vi "Njord Control System.vi"() -> ()   [LabVIEW 2014]
doc: "The main VI"
uses:
  Supervisor/Supervisor.lvclass
  <vilib>/Platform/TimedLoop/XDataNode/timing_clust.ctl
  <vilib>/Platform/TimedLoop/XDataNode/nitl_modes.ctl
  <vilib>/Platform/TimedLoop/XDataNode/wakeup.ctl
  ROV/Vessel(TCPrefs).vi
  <vilib>/FPGAPlugInAG/cRIO-9074/niLvFpga_Open_cRIO-9074.vi
  ROV/Vessel(FPGARef).vi
  Supervisor/Supervisor().vi
  Library/Helping Routines/ReconnectProcedureScalar.vi
  <vilib>/rvi/interface/nirviOpenFPGA/nirviOpenFPGA.xnode
  FPGA Bitfiles/MinervaControlSy_FPGATarget_9870InterfaceDMA_4D1233B8.lvbitx
  cRIO/FPGA/9870 Interface DMA (FPGA).vi
  <vilib>/Platform/TimedLoop/XDataNode/XDataNode.xnode
  Thruster/Thruster.lvclass
  ROV/Vessel.lvclass
  <vilib>/Platform/TimedLoop/XDataNode/XDNodeRunTimeDep.lvlib
  Thrust Allocation/Thrust Allocation.lvclass
panel:
  in  "Recieve UDP PSIMSSB":u16=5113
  in  "Recieve UDP GPGGA":u16=5111
  in  "Recieve Navipac TCP Port":u16=5104
  in  "Recieve ROV TCP Port":u16=5102
  in  "Send Telebuf TCP Port":u16=5100
  in  "Communication control":bool=TRUE
  in  "UDP port":u16=1118
  out "remote address TCP joyst":string
  out "remote address TCP send 1":string
  out "remote address TCP recv":string
  in  "Ignore Semaphore\nTCP Send":bool=TRUE
  in  "Period TCP Thread":i64=50
  out "MainThread timed out":bool
  in  "Main\nTimeOut Limit":i32=-1
  in  "TCP Recv\nTimeOut Limit":i32=25
  in  "TCP Send\nTimeOut Limit":i32=25
  in  "TCP Joyst. \nTimeOut Limit":i32=15
  out "Error TCP Recv":errorcluster
  out "Error TCP Joystick":errorcluster
  out "Error TCP Send":errorcluster
  out "Error MainThread":errorcluster
  in  "Base Port Send TCP":u16=8500
  in  "Port Recv TCP":u16=8510
  in  "Port Joyst.TCP":u16=8520
  out "TCP Joyst. Iteration Duration":u32
  out "TCP Recv Iteration Duration":u32
  out "TCP Recv timed out":bool
  out "TCP Joystick timed out":bool
  out "TCP Send timed out":bool
  out "TCP Send Iteration Duration":i64
  out "TCP Send\nFinished Late?":bool
  out "Main Iteration Duration":i64
  out "Main Thread\nFinished Late?":bool
  out "Exit Error":errorcluster
  in  "Cancel Button":bool
  out "Supervisor":refnum<class "Supervisor.lvclass">
  # "Njord"
  # "cRIO/FPGA"
  # "TCP"
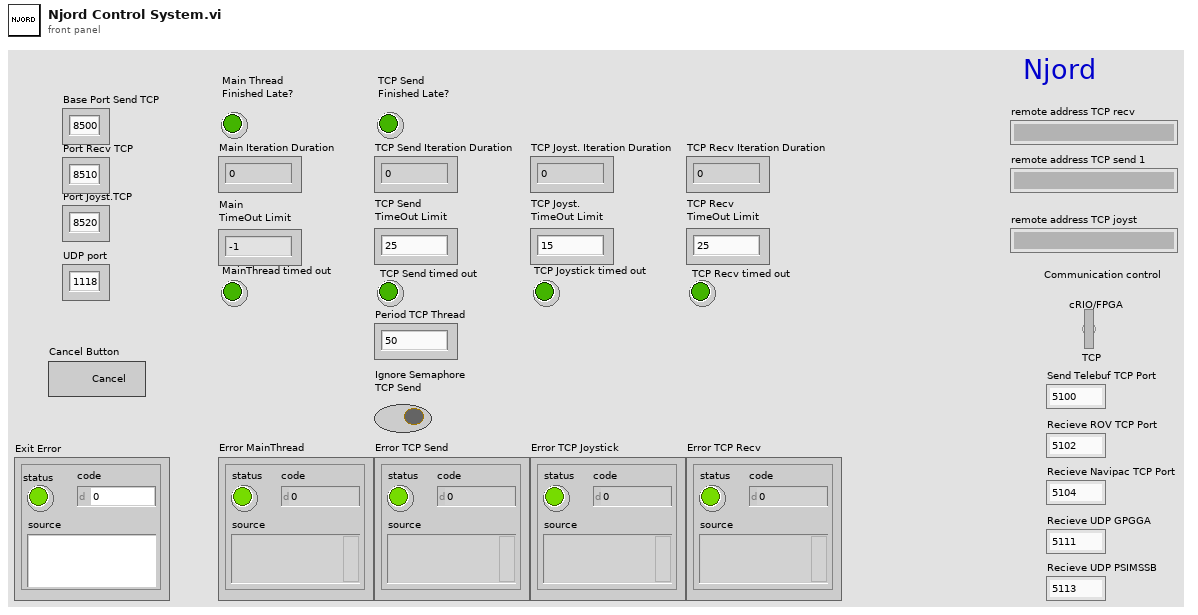
[diagram p1: front panel]
types:
  T1 = typedef "XDNodeRunTimeDep.lvlib/timing_clust.ctl" = cluster{"Expected End [f-1]":u64, "Actual End [f-1]":u64, "Finished Late? [f-1]":bool, "Expected End [i-1]":u64, "Actual End [i-1]":u64, "Finished Late? [i-1]":bool, "Expected Start [i]":u64, "Actual Start [i]":u64, "Expected Start [f]":u64, "Actual Start [f]":u64, "Source Name":string, "Structure Name":string, "Period":i64, "Deadline":i64, "Offset":i64, "Start":i64, "Priority":i32, "Timeout":i32, "Mode":T2, "Wakeup Reason":T3, "Error":errorcluster, "Source Type":string, "Secondary Source Type":string, "Global End Time":u64, "Global Start Time":u64, "Frame Duration":u64, "Iteration Duration":u64, "Assigned CPU":i32, "I/O Scan Engine Mode":u32}
  T2 = typedef "XDNodeRunTimeDep.lvlib/nitl_modes.ctl" = enum32{"No Change", "Process missed periods, maintain original phase", "Discard missed periods, maintain original phase", "Process missed periods, ignore original phase", "Discard missed periods, ignore original phase"}
  T3 = typedef "XDNodeRunTimeDep.lvlib/wakeup.ctl" = enum32{"Normal", "Aborted", "Asynchronous wakeup", "Timing source error", "Timed loop error", "Timeout"}
  T4 = typedef "Semaphore RefNum" = refnum<k1>
  T5 = typedef "Rendezvous RefNum" = refnum<k1>
  T6 = cluster{"Controllers":string[], "Observers":string[]}
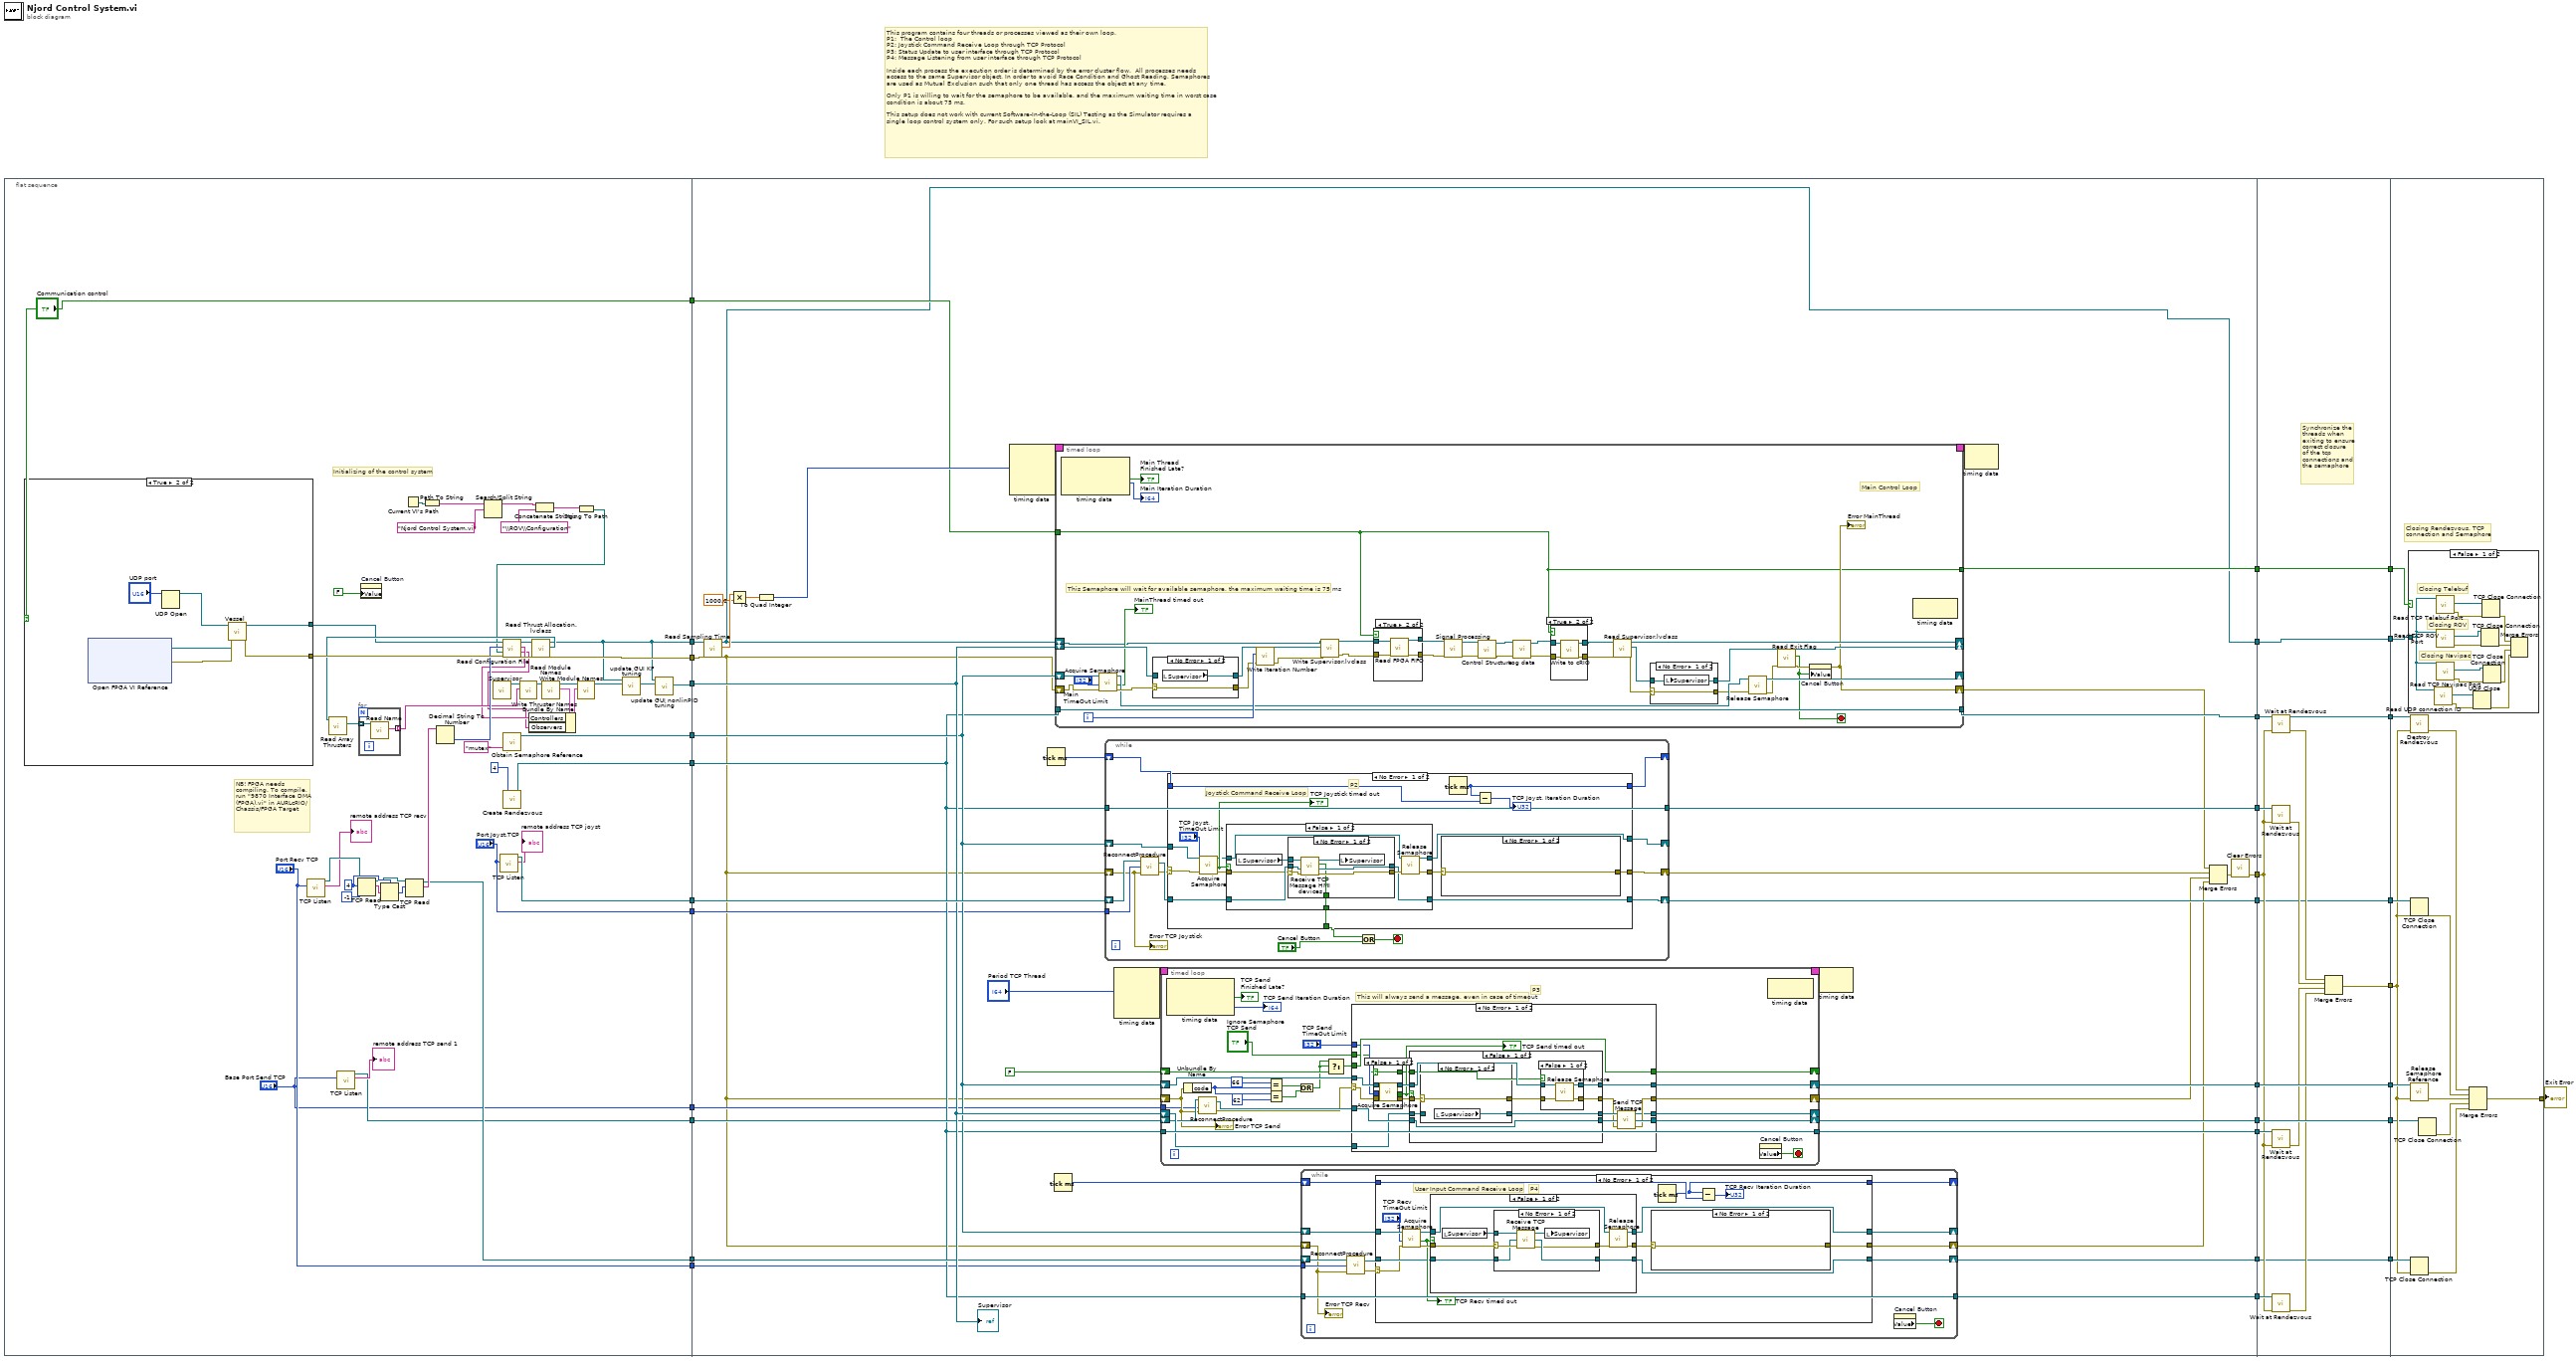
[diagram p0: block diagram]
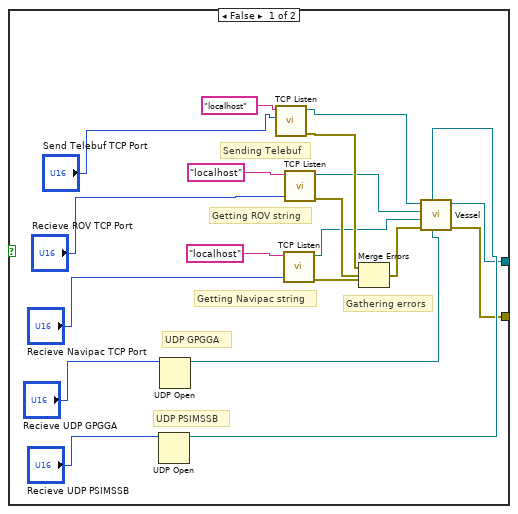
[diagram p2: hidden frame]
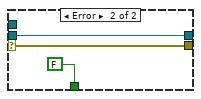
[diagram p3: hidden frame]
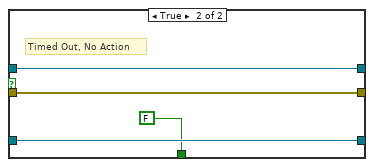
[diagram p4: hidden frame]
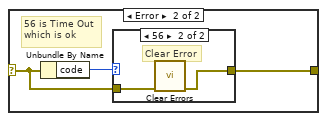
[diagram p5: hidden frame]
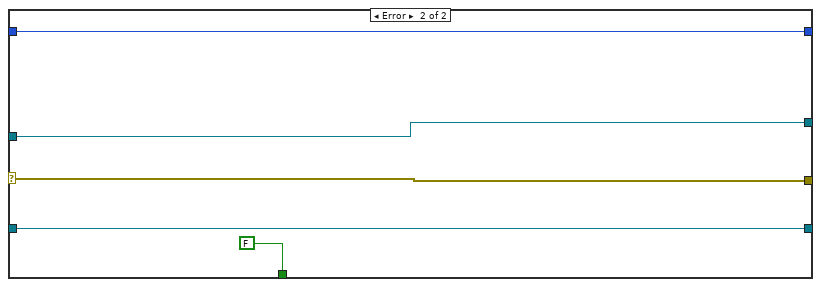
[diagram p7: hidden frame]
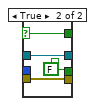
[diagram p8: hidden frame]
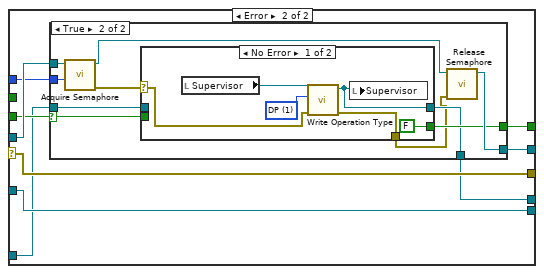
[diagram p12: hidden frame]
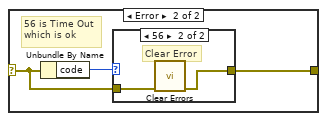
[diagram p15: hidden frame]
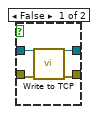
[diagram p20: hidden frame]
diagram:
  # "This program contains four threads or processes viewed as their own loop.\nP1:  The Control loop\nP2: Joystick Command Receive Loop through TCP Protocol\nP3: Status Update to user interface through TCP Protocol\nP4: Message Listening from user interface through TCP Protocol\n\nInside each process the execution order is determined by the error cluster flow.  All processes needs \naccess to the same Supervisor object. In order to avoid Race Condition and Ghost Reading, Semaphores\nare used as Mutual Exclusion such that only one thread has access the object at any time. \n\nOnly P1 is willing to wait for the semaphore to be available, and the maximum waiting time in worst case \ncondition is about 75 ms. \n\nThis setup does not work with current Software-In-the-Loop (SIL) Testing as the Simulator requires a\nsingle loop control system only. For such setup look at mainVI_SIL.vi."
  n1 = flat-sequence {
    tunnel: [w34] -> w32
    tunnel: [w53] -> w31
    tunnel: [w35] -> w30
    tunnel: [w69] -> w29
    tunnel: [w67] -> w28
    tunnel: [w80] -> w27
    tunnel: [w60] -> w22
    tunnel: [w77] -> w16
    tunnel: ["Port Joyst.TCP"] -> w7
    tunnel: ["Base Port Send TCP"] -> w6
    tunnel: ["Port Recv TCP"] -> w5
    tunnel: ["Communication control"] -> w4
    tunnel: w32 -> [w141]
    tunnel: w31 -> [w140]
    tunnel: w30 -> [w139]
    tunnel: w29 -> [w138]
    tunnel: w28 -> [w147]
    tunnel: w27 -> [w136]
    tunnel: [w115] -> w26
    tunnel: [w146] -> w25
    tunnel: [w145] -> w24
    tunnel: [w144] -> w23
    tunnel: w22 -> [w137]
    tunnel: [w135] -> w21
    tunnel: w16 -> [w134]
    tunnel: [w133] -> w15
    tunnel: [w132] -> w14
    tunnel: [w131] -> w13
    tunnel: [w130] -> w12
    tunnel: [w119] -> w10
    tunnel: w7 -> [w123]
    tunnel: w6 -> [w122]
    tunnel: w5 -> [w121]
    tunnel: w4 -> [w117]
    tunnel: [w116] -> w2
    tunnel: w26 -> [w461]
    tunnel: w25 -> [w463]
    tunnel: w24 -> [w475]
    tunnel: w23 -> [w476]
    tunnel: w21 -> [w464]
    tunnel: [w463] -> w20
    tunnel: [w476] -> w19
    tunnel: [w475] -> w18
    tunnel: [w464] -> w17
    tunnel: w15 -> [w474]
    tunnel: w14 -> [w473]
    tunnel: w13 -> [w471]
    tunnel: w12 -> [w472]
    tunnel: [w470] -> w11
    tunnel: w10 -> [w469]
    tunnel: [w462] -> w9
    tunnel: [w461] -> w3
    tunnel: w2 -> [w460]
    tunnel: [w460] -> w1
    tunnel: w20 -> [w490]
    tunnel: w19 -> [w489]
    tunnel: w18 -> [w480]
    tunnel: w17 -> [w488]
    tunnel: w11 -> [w487]
    tunnel: w9 -> [w486]
    tunnel: [w481] -> w8
    tunnel: w3 -> [w478]
    tunnel: w1 -> [w477]
    frame #0 {
      w74 = 4 ("bytes to read")
      # "Initializing of the control system"
      # "NB! FPGA needs compiling. To compile, run \"9870 Interface DMA (FPGA).vi\" in AURLcRIO/Chassis/FPGA Target"
      n2 = case shown="True" "Communication control" {
        tunnel: [w83 w106] -> w79
        tunnel: [w82 w101] -> w45
        frame False {
          # "UDP PSIMSSB"
          # "UDP GPGGA"
          # "Gathering errors"
          # "Sending Telebuf"
          # "Getting Navipac string"
          # "Getting ROV string"
          n3 = UDP Open(11:"Recieve UDP PSIMSSB") -> (port=w86:refnum<k16>)  [unwired: 4 in, 2 out]
          n4 = UDP Open(11:"Recieve UDP GPGGA") -> (port=w85:refnum<k16>)  [unwired: 4 in, 2 out]
          n5 = call <vilib>:"TCP Listen.vi"("port"="Send Telebuf TCP Port", "service name"="localhost") -> ("error out"=w97:errorcluster, "connection ID"=w89:refnum<k5>)  [unwired: 5 in, 3 out]
          n6 = call <vilib>:"TCP Listen.vi"("port"="Recieve Navipac TCP Port", "service name"="localhost") -> ("error out"=w98:errorcluster, "connection ID"=w87:refnum<k5>)  [unwired: 5 in, 3 out]
          n7 = call <vilib>:"TCP Listen.vi"("port"="Recieve ROV TCP Port", "service name"="localhost") -> ("error out"=w99:errorcluster, "connection ID"=w88:refnum<k5>)  [unwired: 5 in, 3 out]
          n8 = Merge Errors(w97, w99, w98) -> (w84:errorcluster)
          n9 = call-poly "Vessel.vi"("UDP GPGGA"=w85, "UDP PSIMSSB"=w86, "error in (no error)"=w84, "TCP Navipac"=w87, "TCP ROV"=w88, "TCP Telebuf"=w89) -> ("error out"=w83:errorcluster, "Vessel.lvclass"=w82:refnum<class "Vessel.lvclass">)  [unwired: 4 in]
        }
        frame True {
          n10 = xnode "Open FPGA VI Reference"() -> ("FPGA VI Reference Out"=w104:refnum<k20>, "error out"=w105:errorcluster)  [unwired: 2 in]
          n11 = UDP Open(11:"UDP port") -> (port=w102:refnum<k16>)  [unwired: 4 in, 2 out]
          n12 = call-poly "Vessel.vi"("error in (no error)"=w105, "FPGA VI Reference"=w104, "UDP connection ID"=w102) -> ("error out"=w106:errorcluster, "Vessel.lvclass"=w101:refnum<class "Vessel.lvclass">)  [unwired: 7 in]
        }
      }
      n13 = call <vilib>:"TCP Listen.vi"("port"="Port Recv TCP") -> ("remote address"=→"remote address TCP recv":string, "connection ID"=w68:refnum<k5>)  [unwired: 6 in, 3 out]
      n14 = call <vilib>:"TCP Listen.vi"("port"="Base Port Send TCP") -> ("remote address"=→"remote address TCP send 1":string, "connection ID"=w60:refnum<k5>)  [unwired: 6 in, 3 out]
      n15 = TCP Read(connection ID=w68, bytes to read=w74, 9:-1 ("timeout ms (25000)")) -> (connection ID out=w72:refnum<k5>, data out=w75:string)  [unwired: 2 in, 1 out]
      n16 = property on="Cancel Button" class="Bool (strict)"("Value"=FALSE) -> ()  [unwired: 2 in, 2 out]
      n17 = Type Cast(type=w74, x=w75) -> (*(type *) &x=w73:i32)
      n18 = Current VI's Path() -> (path=w44:path)
      n19 = TCP Read(connection ID=w72, bytes to read=w73) -> (connection ID out=w69:refnum<k5>, data out=w71:string)  [unwired: 3 in, 1 out]
      n20 = Path To String(path=w44) -> (string=w42:string)
      n21 = Decimal String To Number(string=w71) -> (number=w70:i32)  [unwired: 2 in, 1 out]
      n22 = Search/Split String(string=w42, search string/char (-)="Njord Control System.vi") -> (substring before match=w41:string)  [unwired: 1 in, 2 out]
      n23 = call-poly "Supervisor.vi"() -> ("Supervisor Out"=w57:refnum<class "Supervisor.lvclass">)  [unwired: 11 in]
      n24 = call <vilib>:"TCP Listen.vi"("port"="Port Joyst.TCP") -> ("remote address"=→"remote address TCP joyst":string, "connection ID"=w67:refnum<k5>)  [unwired: 6 in, 3 out]
      n25 = call <vilib>:"Obtain Semaphore Reference.vi"("name (unnamed)"="mutex") -> ("semaphore"=w80:T4)  [unwired: 4 in, 2 out]
      n26 = call <vilib>:"Create Rendezvous.vi"("size (2)"=4) -> ("rendezvous"=w77:T5)  [unwired: 4 in, 2 out]
      n27 = Concatenate Strings(w41, "\\ROV\\Configuration" ("string")) -> (w39:string)
      n28 = String To Path(string=w39) -> (path=w38:path)
      n29 = call "Read Configuration File.vi"("error in (no error)"=w79, "File Path Control"=w38, "ROV Selector"=w70, "Vessel In"=w45) -> ("error out"=w54:errorcluster, "Observer Names"=w46:string[], "Controller Names"=w47:string[], "Vessel Out"=w55:refnum<class "Vessel.lvclass">)  [unwired: 4 in]
      n30 = call "Read Thrust Allocation.lvclass.vi"("error in (no error)"=w54, "Vessel in"=w55) -> ("error out"=w53:errorcluster, "Thrust Allocation.lvclass"=w52:refnum<class "Thrust Allocation.lvclass">, "Vessel out"=w34:refnum<class "Vessel.lvclass">)  [unwired: 7 in]
      n31 = call "Read Array Thrusters.vi"("Thrust Allocation in"=w52) -> ("Array Thrusters"=w58:refnum<class "Thruster.lvclass">[])  [unwired: 8 in, 2 out]
      n32 = for {
        tunnel: w58 -> [w108] mode=indexing
        tunnel: [w107] -> w56 mode=indexing
        n33 = call-dynamic "Read Name.vi"("Thruster in"=w108) -> ("Name"=w107:string)  [unwired: 8 in, 2 out]
      }
      n34 = call-dynamic "Write Thruster Names.vi"("Thruster Names"=w56, "Supervisor in"=w57) -> ("Supervisor out"=w51:refnum<class "Supervisor.lvclass">)  [unwired: 8 in, 1 out]
      n35 = call-dynamic "Read Module Names.vi"("Supervisor in"=w51) -> ("Module Names"=w49:T6, "Supervisor out"=w50:refnum<class "Supervisor.lvclass">)  [unwired: 8 in, 1 out]
      n36 = Bundle By Name(cluster=w49, "Controllers"=w47, "Observers"=w46) -> (w48:T6)
      n37 = call-dynamic "Write Module Names.vi"("Module Names"=w48, "Supervisor in"=w50) -> ("Supervisor out"=w37:refnum<class "Supervisor.lvclass">)  [unwired: 8 in, 1 out]
      n38 = call "update GUI KF tuning.vi"("Supervisor in"=w37, "Vessel in"=w34) -> ("Supervisor"=w36:refnum<class "Supervisor.lvclass">)  [unwired: 9 in]
      n39 = call "update GUI nonlinPID tuning.vi"("Supervisor in"=w36, "Vessel in"=w34) -> ("Supervisor"=w35:refnum<class "Supervisor.lvclass">)  [unwired: 9 in]
    }
    frame #1 {
      n40 = call-dynamic "Read Sampling Time.vi"("error in (no error)"=w140, "Vessel in"=w141) -> ("error out"=w118:errorcluster, "Sampling Time"=w143:dbl, "Vessel out"=w115:refnum<class "Vessel.lvclass">)  [unwired: 7 in]
      n41 = Multiply(x=w143, y=1000.0) -> (x*y=w129:dbl)
      n42 = To Quad Integer(1:w129) -> (0:w128:i64)
      n43 = node-c288(w128) -> (w149:T1)  [unwired: 3 in]
      n44 = Tick Count (ms)() -> (millisecond timer value=w109:u32)
      n45 = Tick Count (ms)() -> (millisecond timer value=w114:u32)
      n46 = timed-loop {
        timing: w149 -> [_]
        timing-out: [_] -> w148
        shift-right: [w425] -> _
        shift-left: w136 -> [w427]
        shift-right: [w423] -> _
        shift-left: w139 -> [w424]
        shift-right: [w407] -> _
        shift-left: w115 -> [w395]
        shift-right: [w404] -> w127
        shift-left: w118 -> [w405]
        tunnel: w134 -> [w415]
        tunnel: [w415] -> w133
        tunnel: w117 -> [w388]
        tunnel: [w388] -> w116
        i -> [w420]
        stop <- w412 stop-if-true
        # "This Semaphore will wait for available semaphore, the maximum waiting time is 75 ms"
        # "Main Control Loop"
        n47 = node-c288() -> (→"Main Thread\nFinished Late?":bool, →"Main Iteration Duration":i64)  [unwired: 1 in, 1 out]
        n48 = call <vilib>:"Acquire Semaphore.vi"("error in (no error)"=w405, "ms timeout (-1)"="Main\nTimeOut Limit", "semaphore"=w427) -> ("error out"=w426:errorcluster, "timed out"=→"MainThread timed out":bool, "semaphore out"=w418:T4)  [unwired: 2 in]
        n49 = case shown="No Error" w426 {
          selector: w426 -> [w448 w451]
          tunnel: [w449 w450] -> w419
          tunnel: [w448 w451] -> w417
          tunnel: w424 -> [_ w450]
          frame No Error {
            n50 = local read "Supervisor"() -> (w449:refnum<class "Supervisor.lvclass">)
          }
          frame Error {
          }
        }
        n51 = call-dynamic "Write Iteration Number.vi"("error in (no error)"=w417, "Iteration Number"=w420, "Supervisor in"=w419) -> ("error out"=w393:errorcluster, "Supervisor out"=w394:refnum<class "Supervisor.lvclass">)  [unwired: 7 in]
        n52 = call "Write Supervisor.lvclass.vi"("error in (no error)"=w393, "Supervisor.lvclass"=w394, "Vessel in"=w395) -> ("error out"=w396:errorcluster, "Vessel out"=w397:refnum<class "Vessel.lvclass">)  [unwired: 7 in]
        n53 = case shown="True" w388 {
          tunnel: [w438 w443] -> w398
          tunnel: w397 -> [w439 w442]
          tunnel: [w436 w441] -> w399
          tunnel: w396 -> [w437 w440]
          frame False {
            n54 = call-dynamic "Read TCP FIFO.vi"("Error In"=w437, "Vessel.lvclass"=w439) -> ("Error Out"=w436:errorcluster, "Vessel.lvclass 2"=w438:refnum<class "Vessel.lvclass">)  [unwired: 6 in]
          }
          frame True {
            n55 = call-dynamic "Read FPGA FIFO.vi"("Error In"=w440, "Vessel.lvclass"=w442) -> ("Error Out"=w441:errorcluster, "Vessel.lvclass 2"=w443:refnum<class "Vessel.lvclass">)  [unwired: 6 in]
          }
        }
        n56 = call-dynamic "Signal Processing.vi"("Vessel in"=w398, "error in (no error)"=w399) -> ("Vessel out"=w403:refnum<class "Vessel.lvclass">, "error out"=w402:errorcluster)  [unwired: 16 in]
        n57 = call "Control Structure.vi"("error in (no error)"=w402, "Vessel in"=w403) -> ("error out"=w400:errorcluster, "Vessel out"=w401:refnum<class "Vessel.lvclass">)  [unwired: 8 in]
        n58 = call "Log data.vi"("error in (no error)"=w400, "Vessel in"=w401) -> ("error out"=w391:errorcluster, "Vessel out"=w392:refnum<class "Vessel.lvclass">)  [unwired: 8 in]
        n59 = case shown="True" w388 {
          tunnel: [w430 w435] -> w390
          tunnel: w392 -> [w431 w434]
          tunnel: w391 -> [w429 w433]
          tunnel: [w428 w432] -> w389
          frame False {
            n60 = call-dynamic "Write to TCP.vi"("error in (no error)"=w429, "Vessel in"=w431) -> ("error out"=w428:errorcluster, "Vessel out"=w430:refnum<class "Vessel.lvclass">)  [unwired: 8 in]
          }
          frame True {
            n61 = call-dynamic "Write to cRIO.vi"("error in (no error)"=w433, "Vessel in"=w434) -> ("error out"=w432:errorcluster, "Vessel out"=w435:refnum<class "Vessel.lvclass">)  [unwired: 8 in]
          }
        }
        n62 = call "Read Supervisor.lvclass.vi"("error in (no error)"=w389, "Vessel in"=w390) -> ("error out"=w416:errorcluster, "Supervisor.lvclass"=w409:refnum<class "Supervisor.lvclass">, "Vessel out"=w407:refnum<class "Vessel.lvclass">)  [unwired: 7 in]
        n63 = case shown="No Error" w416 {
          selector: w416 -> [w445 w447]
          tunnel: w409 -> [w444 w446]
          tunnel: [w445 w447] -> w406
          tunnel: [w444 w446] -> w408
          frame No Error {
            n64 = local write "Supervisor"(w444) -> ()
          }
          frame Error {
          }
        }
        n65 = call <vilib>:"Release Semaphore.vi"("error in (no error)"=w406, "semaphore"=w418) -> ("error out"=w422:errorcluster, "semaphore out"=w425:T4)  [unwired: 4 in]
        n66 = call-dynamic "Read Exit Flag.vi"("error in (no error)"=w422, "Supervisor in"=w408) -> ("error out"=w421:errorcluster, "Exit Flag"=w412:bool, "Supervisor out"=w423:refnum<class "Supervisor.lvclass">)  [unwired: 7 in]
        n67 = property on="Cancel Button" class="Bool (strict)"(error in=w421, "Value"=w412) -> (error out=w404:errorcluster)  [unwired: 1 in, 1 out]
        "Error MainThread" <- w404
        n68 = node-c288() -> ()  [unwired: 1 in, 1 out]
      }
      n69 = while {
        shift-right: [w155] -> w126
        shift-left: w118 -> [w161]
        shift-right: [w154] -> w146
        shift-left: w147 -> [w162]
        shift-right: [w156] -> _
        shift-left: w136 -> [w152]
        tunnel: w134 -> [w164]
        tunnel: [w164] -> w132
        shift-right: [w157] -> _
        shift-left: w109 -> [w158]
        tunnel: w123 -> [w163]
        stop <- w160 stop-if-true
        n70 = call-poly "ReconnectProcedure.vi"("Error In"=w161, "Port Number"=w163, "TCP In"=w162) -> ("Error Out"=w150:errorcluster, "TCP Out"=w151:refnum<k5>)
        n71 = case shown="No Error" w150 {
          selector: w150 -> [w166 w213]
          tunnel: [w177 w213] -> w155
          tunnel: [w175 w211] -> w154
          tunnel: [w172 w212] -> w156
          tunnel: [w171 w214] -> w157
          tunnel: w158 -> [w170 w214]
          tunnel: w152 -> [w168 w212]
          tunnel: w151 -> [w167 w211]
          tunnel: [w165 FALSE] -> w153
          frame No Error {
            # "P2"
            # "Joystick Command Receive Loop"
            n72 = call <vilib>:"Acquire Semaphore.vi"("error in (no error)"=w166, "ms timeout (-1)"="TCP Joyst. \nTimeOut Limit", "semaphore"=w168) -> ("error out"=w179:errorcluster, "timed out"=w178:bool, "semaphore out"=w174:T4)  [unwired: 2 in]
            "TCP Joystick timed out" <- w178
            n73 = case shown="False" w178 {
              tunnel: w167 -> [w188 w201]
              tunnel: [w183 w201] -> w175
              tunnel: w179 -> [w187 w202]
              tunnel: [w184 w202] -> w176
              tunnel: w174 -> [w182 w200]
              tunnel: [w181 w200] -> w172
              tunnel: [w180 FALSE] -> w165
              frame False {
                n74 = local read "Supervisor"() -> (w186:refnum<class "Supervisor.lvclass">)
                n75 = case shown="No Error" w187 {
                  selector: w187 -> [w193 w197]
                  tunnel: [w195 w198] -> w183
                  tunnel: [w194 w197] -> w185
                  tunnel: w188 -> [w192 w198]
                  tunnel: w186 -> [w191 _]
                  tunnel: [w189 FALSE] -> w180
                  frame No Error {
                    n76 = call-dynamic "Receive TCP Message HMI devices.vi"("error in (no error)"=w193, "TCP Joystick Ref In"=w192, "Supervisor in"=w191) -> ("error out"=w194:errorcluster, "TCP Joystick Ref Out"=w195:refnum<k5>, "Exit"=w189:bool, "Supervisor out"=w190:refnum<class "Supervisor.lvclass">)  [unwired: 1 in]
                    n77 = local write "Supervisor"(w190) -> ()
                  }
                  frame Error {
                  }
                }
                n78 = call <vilib>:"Release Semaphore.vi"("error in (no error)"=w185, "semaphore"=w182) -> ("error out"=w184:errorcluster, "semaphore out"=w181:T4)  [unwired: 4 in]
              }
              frame True {
                # "Timed Out, No Action"
              }
            }
            n79 = case shown="No Error" w176 {
              selector: w176 -> [w203 w205]
              tunnel: [w203 w204] -> w177
              frame No Error {
              }
              frame Error {
                # "56 is Time Out\nwhich is ok"
                n80 = Unbundle By Name(w205) -> ("code"=w206:i32)
                n81 = case shown="56" w206 {
                  tunnel: w205 -> [w207 w209]
                  tunnel: [w207 w208] -> w204
                  frame Default {
                  }
                  frame 56 {
                    # "Clear Error"
                    n82 = call <vilib>:"Clear Errors.vi"("error in (no error)"=w209) -> ("error out"=w208:errorcluster)  [unwired: 5 in, 1 out]
                  }
                }
              }
            }
            n83 = Tick Count (ms)() -> (millisecond timer value=w171:u32)
            n84 = Subtract(x=w171, y=w170) -> (x-y=→"TCP Joyst. Iteration Duration":u32)
          }
          frame Error {
          }
        }
        n85 = Or(x=w153, y="Cancel Button") -> (x .or. y?=w160:bool)
        "Error TCP Joystick" <- w161
      }
      n86 = node-c288("Period TCP Thread") -> (w111:T1)  [unwired: 3 in]
      n87 = timed-loop {
        timing: w111 -> [_]
        timing-out: [_] -> w110
        shift-right: [w239] -> w145
        shift-left: w137 -> [w219]
        shift-right: [w240] -> w144
        shift-left: w136 -> [w233]
        shift-right: [w238] -> _
        shift-left: w139 -> [w232]
        shift-right: [w237] -> w125
        shift-left: w118 -> [w216]
        tunnel: w134 -> [w235]
        tunnel: [w235] -> w130
        tunnel: w122 -> [w215]
        shift-right: [w230] -> _
        shift-left: FALSE -> [w224]
        stop <- w236 stop-if-true
        # "P3"
        # "This will always send a message, even in case of timeout"
        n88 = node-c288() -> (→"TCP Send\nFinished Late?":bool, →"TCP Send Iteration Duration":i64)  [unwired: 1 in, 1 out]
        n89 = Unbundle By Name(w216) -> ("code"=w227:i32)
        n90 = call-poly "ReconnectProcedure.vi"("Error In"=w216, "Port Number"=w215, "TCP In"=w219) -> ("Error Out"=w217:errorcluster, "TCP Out"=w218:refnum<k5>)
        n91 = Equal?(x=66, y=w227) -> (x = y?=w226:bool)
        n92 = Equal?(x=w227, y=62) -> (x = y?=w225:bool)
        n93 = Or(x=w226, y=w225) -> (x .or. y?=w223:bool)
        n94 = Select(t=w223, s=w223, f=w224) -> (s? t:f=w222:bool)
        n95 = case shown="No Error" w217 {
          selector: w217 -> [w242 w300]
          tunnel: [w256 w297] -> w240
          tunnel: [w251 w299] -> w239
          tunnel: [w241 w293] -> w238
          tunnel: [w250 w300] -> w237
          tunnel: w233 -> [w249 w298]
          tunnel: w218 -> [w248 w299]
          tunnel: w232 -> [w247 w294]
          tunnel: [w246 w296] -> w230
          tunnel: w222 -> [w246 w295]
          tunnel: "TCP Send\nTimeOut Limit" -> [w245 w292]
          tunnel: "Ignore Semaphore\nTCP Send" -> [w244 _]
          frame No Error {
            n96 = case shown="False" w244 {
              selector: w244 -> [w259 w268]
              tunnel: [w264 w266] -> w258
              tunnel: [w263 w267] -> w257
              tunnel: [w262 FALSE] -> w255
              tunnel: w249 -> [w261 w267]
              tunnel: w245 -> [w260 _]
              tunnel: [w259 w268] -> w243
              tunnel: w242 -> [_ w266]
              frame False {
                n97 = call <vilib>:"Acquire Semaphore.vi"("ms timeout (-1)"=w260, "semaphore"=w261) -> ("error out"=w264:errorcluster, "timed out"=w262:bool, "semaphore out"=w263:T4)  [unwired: 3 in]
              }
              frame True {
              }
            }
            "TCP Send timed out" <- w255
            n98 = case shown="False" w255 {
              tunnel: w258 -> [w277 w288]
              tunnel: w257 -> [w270 w289]
              tunnel: w248 -> [w271 w290]
              tunnel: [w271 w290] -> w254
              tunnel: [w275 w289] -> w256
              tunnel: [w273 w291] -> w253
              tunnel: w247 -> [w274 w291]
              tunnel: [w272 w288] -> w252
              tunnel: w243 -> [w269 _]
              frame False {
                n99 = case shown="No Error" w277 {
                  selector: w277 -> [w284 w287]
                  tunnel: [w285 w286] -> w273
                  tunnel: [w284 w287] -> w276
                  tunnel: w274 -> [_ w286]
                  frame No Error {
                    n100 = local read "Supervisor"() -> (w285:refnum<class "Supervisor.lvclass">)
                  }
                  frame Error {
                  }
                }
                n101 = case shown="False" w269 {
                  tunnel: w276 -> [w281 w282]
                  tunnel: [w280 w283] -> w275
                  tunnel: [w279 w282] -> w272
                  tunnel: w270 -> [w278 w283]
                  frame False {
                    n102 = call <vilib>:"Release Semaphore.vi"("error in (no error)"=w281, "semaphore"=w278) -> ("error out"=w279:errorcluster, "semaphore out"=w280:T4)  [unwired: 4 in]
                  }
                  frame True {
                  }
                }
              }
              frame True {
                # "Time out, no action, use old supervisor"
              }
            }
            n103 = call "Send TCP Message.vi"("Error In"=w252, "TCP Network Connection Refnum"=w254, "Supervisor in"=w253) -> ("Error Out"=w250:errorcluster, "TCP Network Connection Refnum Out"=w251:refnum<k5>, "Supervisor out"=w241:refnum<class "Supervisor.lvclass">)
          }
          frame Error {
            n104 = case shown="True" w295 {
              selector: w295 -> [w303 w309]
              tunnel: w298 -> [w301 w311]
              tunnel: [w301 w310] -> w297
              tunnel: [w303 w308] -> w296
              tunnel: w294 -> [w302 w307]
              tunnel: [w302 w306] -> w293
              tunnel: w292 -> [_ w304]
              frame False {
              }
              frame True {
                n105 = call <vilib>:"Acquire Semaphore.vi"("ms timeout (-1)"=w304, "semaphore"=w311) -> ("error out"=w313:errorcluster, "semaphore out"=w312:T4)  [unwired: 3 in, 1 out]
                n106 = case shown="No Error" w313 {
                  selector: w313 -> [w315 w320]
                  tunnel: w309 -> [_ w321]
                  tunnel: [FALSE w321] -> w308
                  tunnel: w307 -> [_ w322]
                  tunnel: [w317 w322] -> w306
                  tunnel: [w314 w320] -> w305
                  frame No Error {
                    w319 = u16 1 items=["Tracking", "DP", "Joystick"] ("Operation Type")
                    n107 = local read "Supervisor"() -> (w316:refnum<class "Supervisor.lvclass">)
                    n108 = call-dynamic "Write Operation Type.vi"("error in (no error)"=w315, "Operation Type"=w319, "Supervisor in"=w316) -> ("error out"=w314:errorcluster, "Supervisor out"=w317:refnum<class "Supervisor.lvclass">)  [unwired: 7 in]
                    n109 = local write "Supervisor"(w317) -> ()
                  }
                  frame Error {
                  }
                }
                n110 = call <vilib>:"Release Semaphore.vi"("error in (no error)"=w305, "semaphore"=w312) -> ("semaphore out"=w310:T4)  [unwired: 4 in, 1 out]
              }
            }
          }
        }
        n111 = property on="Cancel Button" class="Bool (strict)"() -> ("Value"=w236:bool)  [unwired: 2 in, 2 out]
        n112 = node-c288() -> ()  [unwired: 1 in, 1 out]
        "Error TCP Send" <- w216
      }
      n113 = while {
        shift-right: [w339] -> w135
        shift-left: w138 -> [w334]
        shift-right: [w341] -> w124
        shift-left: w118 -> [w331]
        shift-right: [w340] -> _
        shift-left: w136 -> [w343]
        tunnel: w134 -> [w338]
        tunnel: [w338] -> w131
        shift-right: [w336] -> _
        shift-left: w114 -> [w337]
        tunnel: w121 -> [w332]
        stop <- w342 stop-if-true
        n114 = call-poly "ReconnectProcedure.vi"("Error In"=w331, "Port Number"=w332, "TCP In"=w334) -> ("Error Out"=w335:errorcluster, "TCP Out"=w333:refnum<k5>)
        n115 = case shown="No Error" w335 {
          selector: w335 -> [w344 w384]
          tunnel: w343 -> [w355 w386]
          tunnel: [w351 w384] -> w341
          tunnel: [w350 w386] -> w340
          tunnel: [w349 w385] -> w339
          tunnel: w337 -> [w348 w387]
          tunnel: [w347 w387] -> w336
          tunnel: w333 -> [w345 w385]
          frame No Error {
            # "P4"
            # "User Input Command Receive Loop"
            n116 = call <vilib>:"Acquire Semaphore.vi"("error in (no error)"=w344, "ms timeout (-1)"="TCP Recv\nTimeOut Limit", "semaphore"=w355) -> ("error out"=w357:errorcluster, "timed out"=w356:bool, "semaphore out"=w354:T4)  [unwired: 2 in]
            "TCP Recv timed out" <- w356
            n117 = case shown="False" w356 {
              tunnel: [w367 w383] -> w352
              tunnel: [w372 w382] -> w349
              tunnel: w345 -> [w369 w382]
              tunnel: w357 -> [w371 w383]
              tunnel: w354 -> [w366 w381]
              tunnel: [w365 w381] -> w350
              frame False {
                n118 = local read "Supervisor"() -> (w370:refnum<class "Supervisor.lvclass">)
                n119 = case shown="No Error" w371 {
                  selector: w371 -> [w378 w380]
                  tunnel: [w373 w380] -> w368
                  tunnel: w370 -> [w377 _]
                  tunnel: [w376 w379] -> w372
                  tunnel: w369 -> [w375 w379]
                  frame No Error {
                    n120 = call "Receive TCP Message.vi"("Error In"=w378, "TCP Network Connection Refnum"=w375, "Supervisor In"=w377) -> ("Error Out"=w373:errorcluster, "TCP Network Connection Refnum Out"=w376:refnum<k5>, "Supervisor Out"=w374:refnum<class "Supervisor.lvclass">)
                    n121 = local write "Supervisor"(w374) -> ()
                  }
                  frame Error {
                  }
                }
                n122 = call <vilib>:"Release Semaphore.vi"("error in (no error)"=w368, "semaphore"=w366) -> ("error out"=w367:errorcluster, "semaphore out"=w365:T4)  [unwired: 4 in]
              }
              frame True {
                # "Time Out, No Action"
              }
            }
            n123 = case shown="No Error" w352 {
              selector: w352 -> [w358 w360]
              tunnel: [w358 w359] -> w351
              frame No Error {
              }
              frame Error {
                # "56 is Time Out\nwhich is ok"
                n124 = Unbundle By Name(w360) -> ("code"=w361:i32)
                n125 = case shown="56" w361 {
                  tunnel: w360 -> [w362 w364]
                  tunnel: [w362 w363] -> w359
                  frame Default {
                  }
                  frame 56 {
                    # "Clear Error"
                    n126 = call <vilib>:"Clear Errors.vi"("error in (no error)"=w364) -> ("error out"=w363:errorcluster)  [unwired: 5 in, 1 out]
                  }
                }
              }
            }
            n127 = Tick Count (ms)() -> (millisecond timer value=w347:u32)
            n128 = Subtract(x=w347, y=w348) -> (x-y=→"TCP Recv Iteration Duration":u32)
          }
          frame Error {
          }
        }
        n129 = property on="Cancel Button" class="Bool (strict)"() -> ("Value"=w342:bool)  [unwired: 2 in, 2 out]
        "Error TCP Recv" <- w331
      }
      n130 = node-c288(w110) -> ()  [unwired: 1 out]
      n131 = node-c288(w148) -> ()  [unwired: 1 out]
      n132 = Merge Errors(w127, w126, w125, w124) -> (w120:errorcluster)
      n133 = call <vilib>:"Clear Errors.vi"("error in (no error)"=w120) -> ("error out"=w119:errorcluster)  [unwired: 5 in, 1 out]
      "Supervisor" <- w139
    }
    frame #2 {
      # "Synchronize the\nthreads when \nexiting to ensure\ncorrect closure\nof the tcp \nconnections and\nthe semaphore"
      n134 = call <vilib>:"Wait at Rendezvous.vi"("error in (no error)"=w469, "rendezvous"=w474) -> ("error out"=w468:errorcluster, "rendezvous out"=w470:T5)  [unwired: 3 in, 1 out]
      n135 = call <vilib>:"Wait at Rendezvous.vi"("error in (no error)"=w469, "rendezvous"=w473) -> ("error out"=w467:errorcluster)  [unwired: 3 in, 2 out]
      n136 = call <vilib>:"Wait at Rendezvous.vi"("error in (no error)"=w469, "rendezvous"=w472) -> ("error out"=w466:errorcluster)  [unwired: 3 in, 2 out]
      n137 = call <vilib>:"Wait at Rendezvous.vi"("error in (no error)"=w469, "rendezvous"=w471) -> ("error out"=w465:errorcluster)  [unwired: 3 in, 2 out]
      n138 = Merge Errors(w468, w467, w466, w465) -> (w462:errorcluster)
    }
    frame #3 {
      # "Closing Rendezvous, TCP \nconnection and Semaphore"
      n139 = case shown="False" w477 {
        tunnel: w478 -> [w500 _]
        frame False {
          # "Closing Navipac"
          # "Closing ROV"
          # "Closing Telebuf"
          n140 = call-dynamic "Read UDP connection ID.vi"("Vessel in"=w500) -> ("error out"=w495:errorcluster, "UDP connection ID"=w499:refnum<k16>)  [unwired: 8 in, 1 out]
          n141 = call-dynamic "Read TCP Telebuf Port.vi"("Vessel in"=w500) -> ("error out"=w498:errorcluster, "TCP Network Connection Refnum"=w503:refnum<k5>)  [unwired: 8 in, 1 out]
          n142 = call-dynamic "Read TCP ROV Port.vi"("Vessel in"=w500) -> ("error out"=w497:errorcluster, "TCP Network Connection Refnum"=w502:refnum<k5>)  [unwired: 8 in, 1 out]
          n143 = call-dynamic "Read TCP Navipac Port.vi"("Vessel in"=w500) -> ("error out"=w496:errorcluster, "TCP Network Connection Refnum"=w501:refnum<k5>)  [unwired: 8 in, 1 out]
          n144 = UDP Close(connection ID=w499, 8:w495) -> (error out=w491:errorcluster)  [unwired: 1 out]
          n145 = TCP Close Connection(connection ID=w502, error in (no error)=w497) -> (error out=w493:errorcluster)  [unwired: 1 in, 1 out]
          n146 = TCP Close Connection(connection ID=w503, error in (no error)=w498) -> (error out=w494:errorcluster)  [unwired: 1 in, 1 out]
          n147 = TCP Close Connection(connection ID=w501, error in (no error)=w496) -> (error out=w492:errorcluster)  [unwired: 1 in, 1 out]
          n148 = Merge Errors(w494, w493, w492, w491) -> ()  [unwired: 1 out]
        }
        frame True {
        }
      }
      n149 = call <vilib>:"Destroy Rendezvous.vi"("error in (no error)"=w486, "rendezvous"=w487) -> ("error out"=w485:errorcluster)  [unwired: 4 in, 1 out]
      n150 = TCP Close Connection(connection ID=w490, error in (no error)=w486) -> (error out=w484:errorcluster)  [unwired: 1 in, 1 out]
      n151 = call <vilib>:"Release Semaphore Reference.vi"("error in (no error)"=w486, "semaphore"=w489) -> ("error out"=w483:errorcluster)  [unwired: 8 in, 1 out]
      n152 = TCP Close Connection(connection ID=w488, error in (no error)=w486) -> (error out=w482:errorcluster)  [unwired: 1 in, 1 out]
      n153 = TCP Close Connection(connection ID=w480) -> (error out=w479:errorcluster)  [unwired: 2 in, 1 out]
      n154 = Merge Errors(w485, w484, w483, w479, w482) -> (w481:errorcluster)
    }
  }
  "Exit Error" <- w8
